vi "Enqueue Message (same to all queues).vi"(6 "Priority":bool, 7 "Exclude":string, 8 "error in (no error)":errorcluster, 9 "Message Data Array":variant[](array[variant]), 10 "Message":string, 11 "Message Queues in":T1) -> (0 "error out":errorcluster, 3 "Message Queues out":T1)   [LabVIEW 2017, in "Message Queue.lvlib"]
uses:
  All Message Queues.ctl
  Message Cluster.ctl
  Message Queue.lvlib
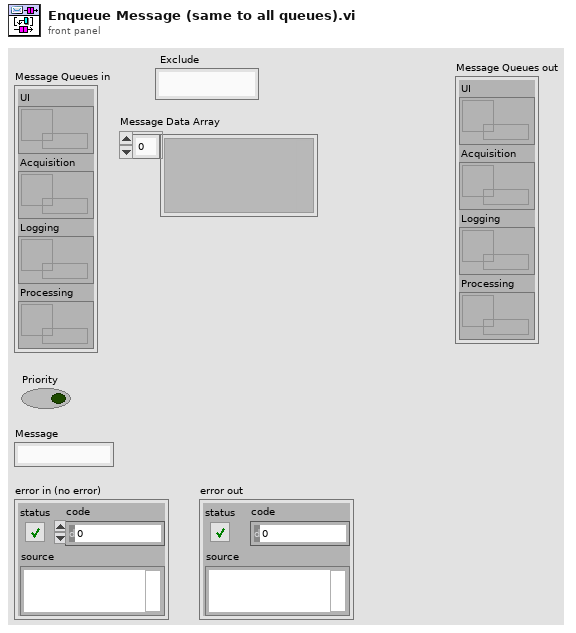
[diagram p1: front panel]
types:
  T1 = typedef "Message Queue.lvlib/All Message Queues.ctl" = cluster{"UI":refnum<queue>, "Acquisition":refnum<queue>, "Logging":refnum<queue>, "Processing":refnum<queue>}
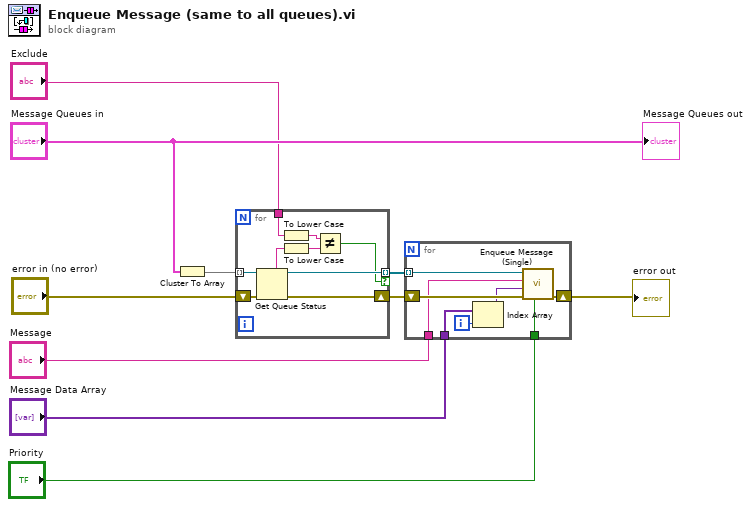
[diagram p0: block diagram]
diagram:
  n1 = Cluster To Array(cluster="Message Queues in") -> (array=w7:refnum<queue>[])
  n2 = for {
    tunnel: w7 -> [w19] mode=indexing
    tunnel: [w18] -> w8 mode=indexing if=w11
    shift-right: [w17] -> w9
    shift-left: "error in (no error)" -> [w16]
    tunnel: "Exclude" -> [w12]
    n3 = Get Queue Status(queue=w19, error in (no error)=w16) -> (queue out=w18:refnum<queue>, queue name=w15:string, error out=w17:errorcluster)  [unwired: 1 in, 5 out]
    n4 = To Lower Case(string=w12) -> (all lower case string=w13:string)
    n5 = To Lower Case(string=w15) -> (all lower case string=w14:string)
    n6 = Not Equal?(x=w13, y=w14) -> (x != y?=w11:bool)
  }
  n7 = for {
    shift-right: [w26] -> w5
    shift-left: w9 -> [w27]
    tunnel: w8 -> [w25] mode=indexing
    tunnel: "Message" -> [w24]
    tunnel: "Priority" -> [w23]
    tunnel: "Message Data Array" -> [w20]
    i -> [w21]
    n8 = Index Array(array=w20, index=w21) -> (element=w22:variant)
    n9 = call "Enqueue Message (Single).vi"("Priority Message? (F)"=w23, "error in (no error)"=w27, "Message Data"=w22, "Message"=w24, "Message Queue"=w25) -> ("error out"=w26:errorcluster)  [unwired: 5 in, 1 out]
  }
  "error out" <- w5
  "Message Queues out" <- "Message Queues in"
